vi "Set Final Column.vi"(8 "error in (no error)":errorcluster, 11 "CCDCamera in":refnum<class "CCDCamera.lvclass">) -> (0 "error out":errorcluster, 3 "CCDCamera out":refnum<class "CCDCamera.lvclass">)   [LabVIEW 2018]
uses:
  CCDCamera.lvclass
  Simulated_CCD_Camera/Simulated_CCD_Camera.lvclass
  C:/Users/observer/Desktop/SPARC4_ACS/SPARC4_ACS/Simulated_CCD_Camera/Simulated_CCD_Camera.lvclass
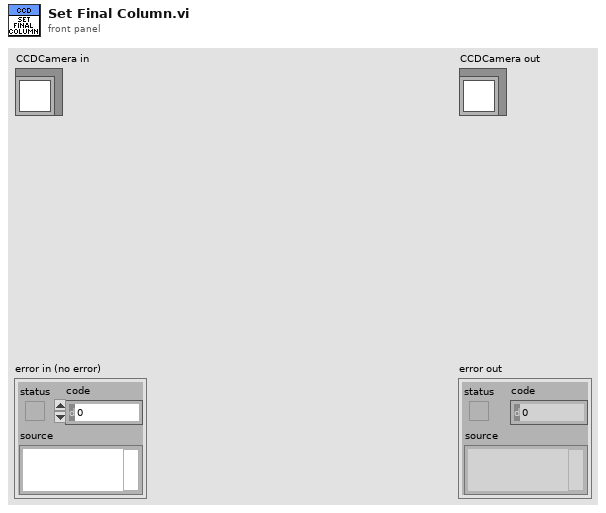
[diagram p1: front panel]
types:
  T1 = cluster{"PREAMP":u16, "READOUT_RATE":u16, "EM_GAIN":u16, "VERTICAL_SHIFT_SPEED":u16, "READ_MODE":u16, "FRAME_TRANSFER":bool, "VERTICAL_CLOCK_VOLTAGE":u16, "ACQUISITION_MODE":u16, "AD_CHANNEL":u16, "EM_MODE":u16, "SHUTTER_TTL":u16, "SHUTTER_OPENING_TIME":u16, "SHUTTER_CLOSING_TIME":u16, "SHUTTER_MODE":u16, "TRIGGER_MODE":u16, "VBIN":u16, "INITIAL_LINE":u16, "INITIAL_COLUMN":u16, "FINAL_LINE":u16, "FINAL_COLUMN":u16, "HBIN":u16}
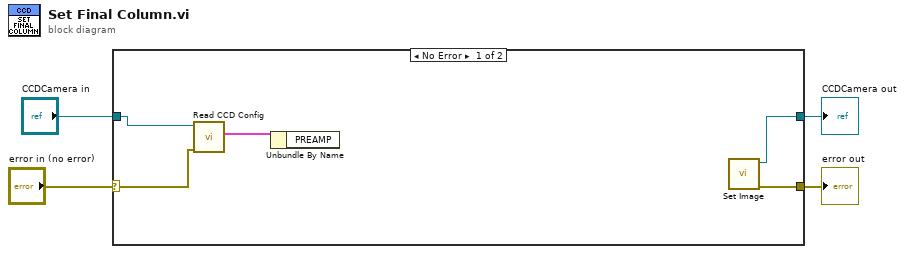
[diagram p0: block diagram]
diagram:
  n1 = case shown="No Error" "error in (no error)" {
    selector: "error in (no error)" -> [w6 w11]
    tunnel: [w9 w11] -> w1
    tunnel: [w8 w10] -> w2
    tunnel: "CCDCamera in" -> [w7 w10]
    frame No Error {
      n2 = call "Read CCD Config.vi"("error in (no error)"=w6, "CCDCamera in"=w7) -> ("CCD Config"=w5:T1)  [unwired: 7 in, 2 out]
      n3 = Unbundle By Name(w5) -> ()  [unwired: 1 out]
      n4 = call-dynamic "Set Image.vi"() -> ("error out"=w9:errorcluster, "CCDCamera out"=w8:refnum<class "CCDCamera.lvclass">)  [unwired: 10 in]
    }
    frame Error {
    }
  }
  "error out" <- w1
  "CCDCamera out" <- w2
